vi "Configure.vi"(8 "error in (no error)":errorcluster, 10 "Parameters":variant, 11 "Output Process in":refnum<class "Sine Process.lvclass">) -> (0 "error out":errorcluster, 3 "Output Process out":refnum<class "Sine Process.lvclass">)   [LabVIEW 2019, in "TimingDRV Engine.lvlib" / "Sine Process.lvclass"]
uses:
  Sine Process.lvclass
  Sine Process.lvclass/Sine Process.ctl
  Parent Classes/Process/Process.lvclass
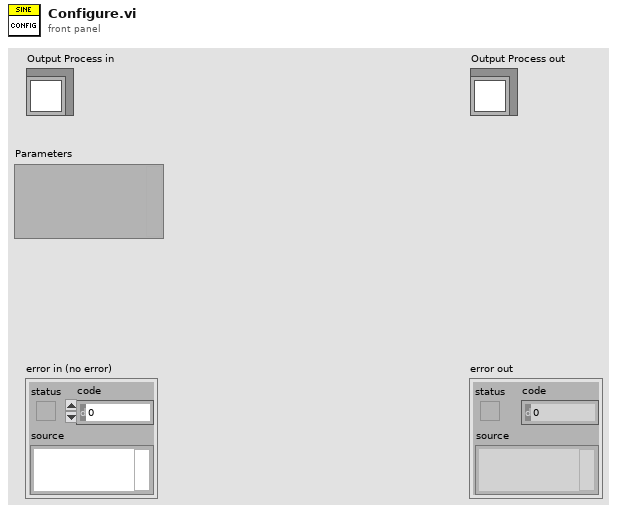
[diagram p1: front panel]
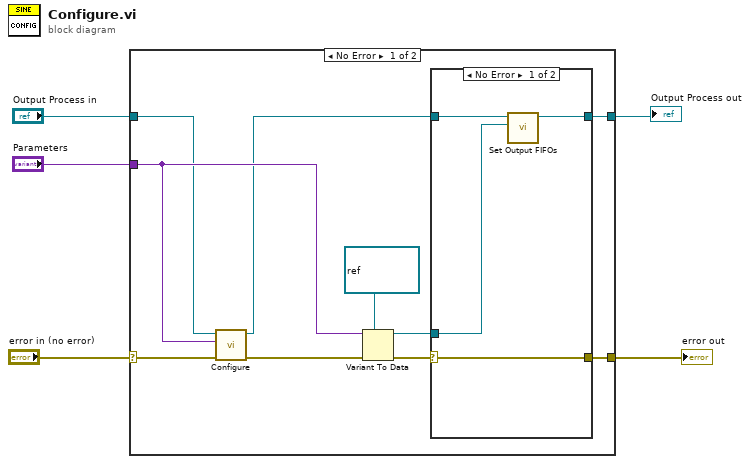
[diagram p0: block diagram]
diagram:
  n1 = case shown="No Error" "error in (no error)" {
    selector: "error in (no error)" -> [w6 w23]
    tunnel: "Parameters" -> [w12 _]
    tunnel: "Output Process in" -> [w10 w22]
    tunnel: [w8 w22] -> w3
    tunnel: [w7 w23] -> w2
    frame No Error {
      n2 = call-parent "Configure.vi"("error in (no error)"=w6, "Parameters"=w12, "Process in"=w10) -> ("error out"=w11:errorcluster, "Process out"=w9:refnum<class "Sine Process.lvclass">)  [unwired: 7 in]
      n3 = Variant To Data(error in=w11, type=refnum<k33> refnum ("Device Outputs FIFO"), Variant=w12) -> (data=w13:refnum<k33>, error out=w14:errorcluster)
      n4 = case shown="No Error" w14 {
        selector: w14 -> [w16 w21]
        tunnel: w9 -> [w19 w20]
        tunnel: w13 -> [w18 _]
        tunnel: [w17 w20] -> w8
        tunnel: [w16 w21] -> w7
        frame No Error {
          n5 = call "Set Output FIFOs.vi"("Output FIFOs"=w18, "Output Process in"=w19) -> ("Output Process out"=w17:refnum<class "Sine Process.lvclass">)  [unwired: 9 in]
        }
        frame Error {
        }
      }
    }
    frame Error {
    }
  }
  "error out" <- w2
  "Output Process out" <- w3
